vi "Finish.vi"   [LabVIEW 2017]
doc: "This VI is called just before exiting. It is expected to close I/O refnum, save collected data, etc."
uses:
  HuskieBoard.ctl
types:
  T1 = typedef "HuskieBoard.ctl" = enum16{"HuskieBoard"}
  T2 = typedef "WPI_SerialPortRef.ctl" = cluster{"DevStatus":errorcluster, "Serial Port Name":refnum<visa-resource-name>}
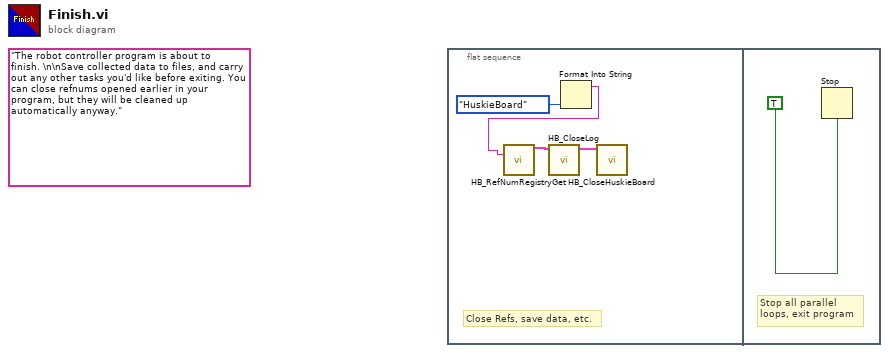
[diagram p0: block diagram]
diagram:
  (unwired) "The robot controller program is about to finish. \n\nSave collected data to files, and carry out any other tasks you'd like before exiting. You can close refnums opened earlier in your program, but they will be cleaned up automatically anyway."
  n1 = flat-sequence {
    frame #0 {
      # "Close Refs, save data, etc."
      n2 = Format Into String(HuskieBoard."HuskieBoard" ("Enum")) -> (resulting string=w2:string)  [unwired: 3 in, 1 out]
      n3 = call <vilib>:"HB_RefNumRegistryGet.vi"("refnum name"=w2) -> ("HBDevRef"=w4:T2)  [unwired: 13 in, 1 out]
      n4 = call <vilib>:"HB_CloseLog.vi"("HBDeviceRef"=w4) -> ("HBDeviceRef"=w1:T2)  [unwired: 9 in, 1 out]
      n5 = call <vilib>:"HB_CloseHuskieBoard.vi"("HBDeviceRef"=w1) -> ()  [unwired: 10 in, 1 out]
    }
    frame #1 {
      # "Stop all parallel\nloops, exit program"
      n6 = Stop(stop? (T)=TRUE ("Quit")) -> ()
    }
  }
